vi "NormalizeArray.vi"(1 "index":i32=1, 2 "Array":dbl[](array[numeric])) -> (0 "x/y":dbl[](array[numeric]))   [LabVIEW 2015]
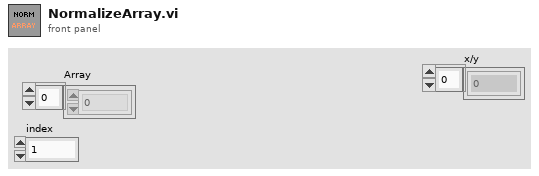
[diagram p1: front panel]
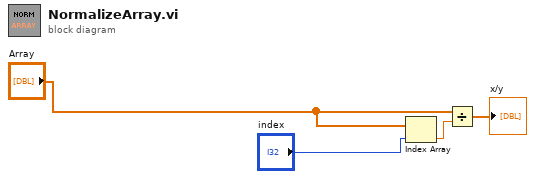
[diagram p0: block diagram]
diagram:
  n1 = Index Array(array="Array", index="index") -> (element=w3:dbl)
  n2 = Divide(x="Array", y=w3) -> (x/y=→"x/y":dbl[])
